vi "Read Configuration.vi"(8 "error in (no error)":errorcluster, 11 "Thermocouple in":refnum<class "Thermocouple.lvclass">) -> (0 "error out":errorcluster, 2 "Configuration":refnum<class "Configuration.lvclass">, 3 "Thermocouple out":refnum<class "Thermocouple.lvclass">)   [LabVIEW 2018, in "Thermocouple.lvlib" / "Thermocouple.lvclass"]
uses:
  Thermocouple.lvclass
  PPLs/Configuration/Configuration.lvlibp/Configuration.lvclass
  Thermocouple.lvclass/Thermocouple.ctl
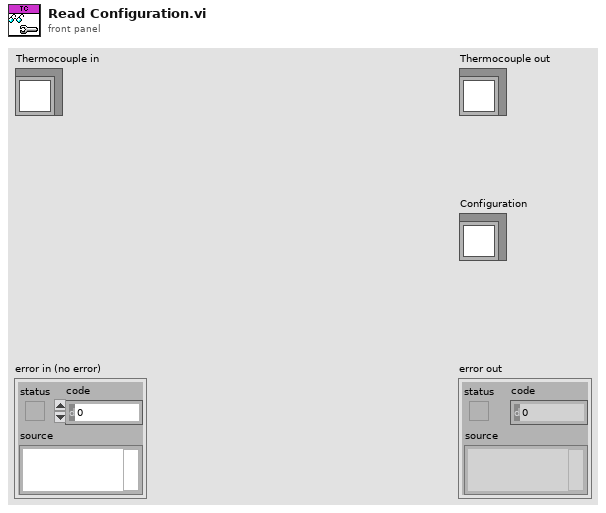
[diagram p1: front panel]
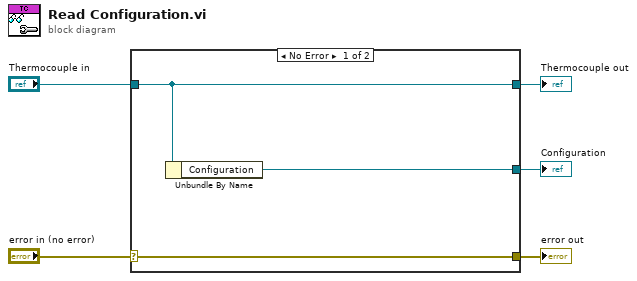
[diagram p0: block diagram]
diagram:
  n1 = case shown="No Error" "error in (no error)" {
    selector: "error in (no error)" -> [w8 w9]
    tunnel: [w8 w9] -> w4
    tunnel: [w7 w10] -> w2
    tunnel: "Thermocouple in" -> [w7 w10]
    tunnel: [w6 _] -> w1
    frame No Error {
      n2 = Unbundle By Name(w7) -> ("Configuration"=w6:refnum<class "Configuration.lvclass">)
    }
    frame Error {
    }
  }
  "error out" <- w4
  "Thermocouple out" <- w2
  "Configuration" <- w1
